vi "GET_DATA.vi"(5 "ulValue":u32=50, 11 "error in (no error)":errorcluster) -> (4 "function return":string, 10 "BytePtr":u8[](array[numeric]), 15 "error out":errorcluster)   [LabVIEW 2017, in "ZBOX_IS.lvlib"]
uses:
  ZBOX_IS.lvlib
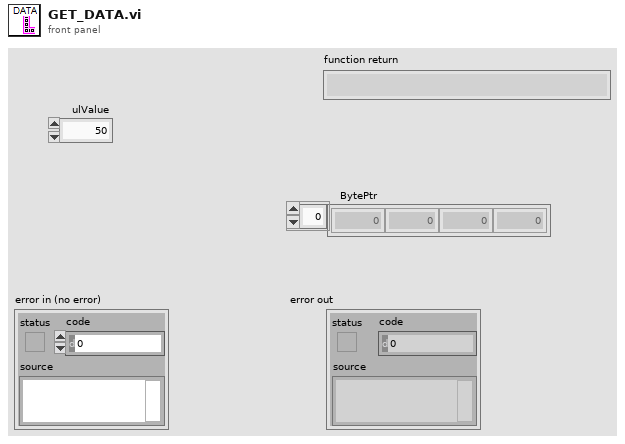
[diagram p1: front panel]
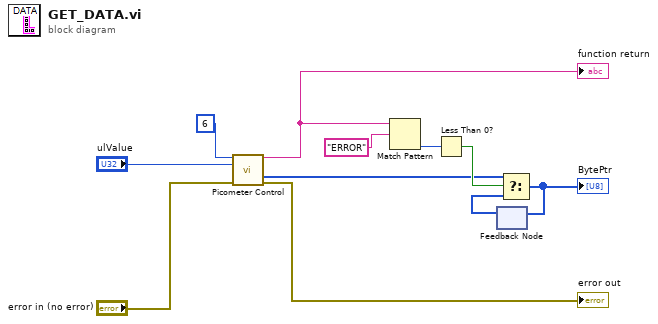
[diagram p0: block diagram]
diagram:
  n1 = call "Picometer Control.vi"("Cmd"=u8 6, "ulValue"="ulValue", "error in (no error)"="error in (no error)") -> ("function return"=w7:string, "BytePtr"=w3:u8[], "error out"=→"error out":errorcluster)  [unwired: 8 in, 2 out]
  "function return" <- w7
  n2 = Match Pattern(string=w7, regular expression="ERROR") -> (offset past match=w5:i32)  [unwired: 1 in, 3 out]
  n3 = Less Than 0?(x=w5) -> (x < 0?=w4:bool)
  n4 = feedback #1() -> (w1:u8[])  [unwired: 1 in]
  n5 = Select(t=w3, s=w4, f=w1) -> (s? t:f=w2:u8[])
  "BytePtr" <- w2
  n6 = feedback-in #1(w2) -> ()
